vi "Email (SubVI).vi"(1 "Subject":string, 2 "Body":string, 3 "Attachment Path":path, 6 "userName":string="DDUSmartHome@gmail.com", 8 "password":string="123qwe_asd", 9 "Recipients Name":string="DDUSmartHome", 10 "Sender's Name":string="DDUSmartHome", 11 "Recipients address":string="DDUSmartHome@gmail.com", 12 "Sender's address":string="DDUSmartHome@gmail.com") -> ()   [LabVIEW 2015]
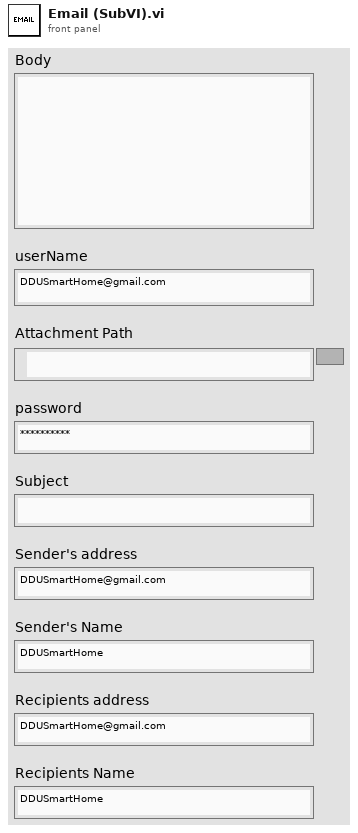
[diagram p1: front panel]
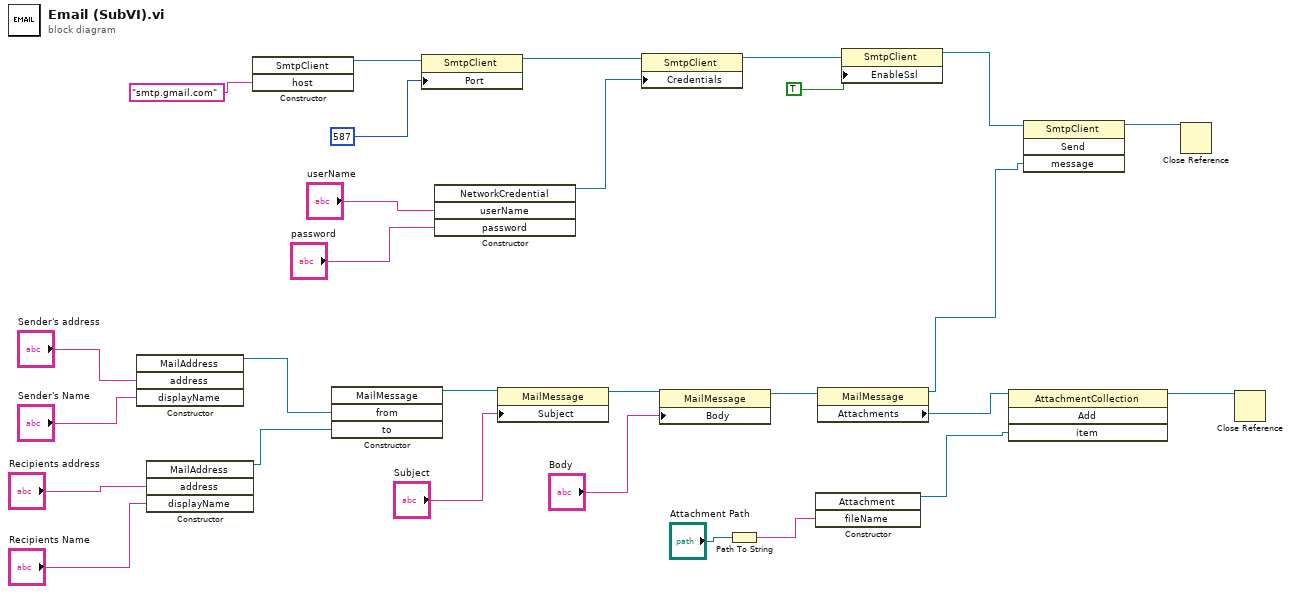
[diagram p0: block diagram]
diagram:
  n1 = constructor class="MailAddress"("address"="Sender's address", "displayName"="Sender's Name") -> (reference out=w6:refnum<k24>)  [unwired: 3 in, 4 out]
  n2 = constructor class="MailAddress"("address"="Recipients address", "displayName"="Recipients Name") -> (reference out=w5:refnum<k24>)  [unwired: 3 in, 4 out]
  n3 = constructor class="SmtpClient"("host"="smtp.gmail.com") -> (reference out=w18:refnum<k24>)  [unwired: 3 in, 3 out]
  n4 = constructor class="MailMessage"("from"=w6, "to"=w5) -> (reference out=w7:refnum<k24>)  [unwired: 3 in, 4 out]
  n5 = property class="SmtpClient"(reference=w18, "Port"=587) -> (reference out=w22:refnum<k24>)  [unwired: 1 in, 1 out]
  n6 = constructor class="NetworkCredential"("userName"="userName", "password"="password") -> (reference out=w23:refnum<k24>)  [unwired: 3 in, 4 out]
  n7 = property class="MailMessage"(reference=w7, "Subject"="Subject") -> (reference out=w9:refnum<k24>)  [unwired: 1 in, 1 out]
  n8 = property class="SmtpClient"(reference=w22, "Credentials"=w23) -> (reference out=w24:refnum<k24>)  [unwired: 1 in, 1 out]
  n9 = property class="MailMessage"(reference=w9, "Body"="Body") -> (reference out=w11:refnum<k24>)  [unwired: 1 in, 1 out]
  n10 = Path To String(path="Attachment Path") -> (string=w13:string)
  n11 = constructor class="Attachment"("fileName"=w13) -> (reference out=w15:refnum<k24>)  [unwired: 3 in, 3 out]
  n12 = property class="MailMessage"(reference=w11) -> (reference out=w27:refnum<k24>, "Attachments"=w14:refnum<k24>)  [unwired: 1 in, 1 out]
  n13 = property class="SmtpClient"(reference=w24, "EnableSsl"=TRUE) -> (reference out=w26:refnum<k24>)  [unwired: 1 in, 1 out]
  n14 = invoke class="AttachmentCollection" method="Add"(reference=w14, "item"=w15) -> (reference out=w16:refnum<k24>)  [unwired: 2 in, 3 out]
  n15 = invoke class="SmtpClient" method="Send"(reference=w26, "message"=w27) -> (reference out=w28:refnum<k24>)  [unwired: 2 in, 3 out]
  n16 = Close Reference(reference=w28) -> ()  [unwired: 1 in, 1 out]
  n17 = Close Reference(reference=w16) -> ()  [unwired: 1 in, 1 out]
